vi "SignalSimulator.vi"() -> (3 "Array":dbl[](array[numeric]))   [LabVIEW 2020]
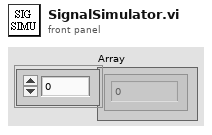
[diagram p1: front panel]
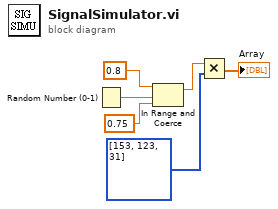
[diagram p0: block diagram]
diagram:
  n1 = Random Number (0-1)() -> (number: 0 to 1=w3:dbl)
  n2 = In Range and Coerce(upper limit=0.8, x=w3, lower limit=0.75) -> (coerced(x)=w4:dbl)  [unwired: 1 out]
  n3 = Multiply(x=w4, y=i32[] [153, 123, 31]) -> (x*y=→"Array":dbl[])
